vi "create.orderbook.commands.for.testing.vi"(11 "OrderBook.Commands.in":T1[](array[typedef]) {"Side (U8)" format="%.0x"; "Order Id (U64)" format="%.0x"; "Symbol (U64)" format="%.0x"}) -> (3 "Words.Out":u64[](array[numeric]) format="%.0x")   [LabVIEW 2022 SP3]
uses:
  arty/orderbook/orderbook.command.ctl
  arty/orderbook/orderbook.command.type.ctl
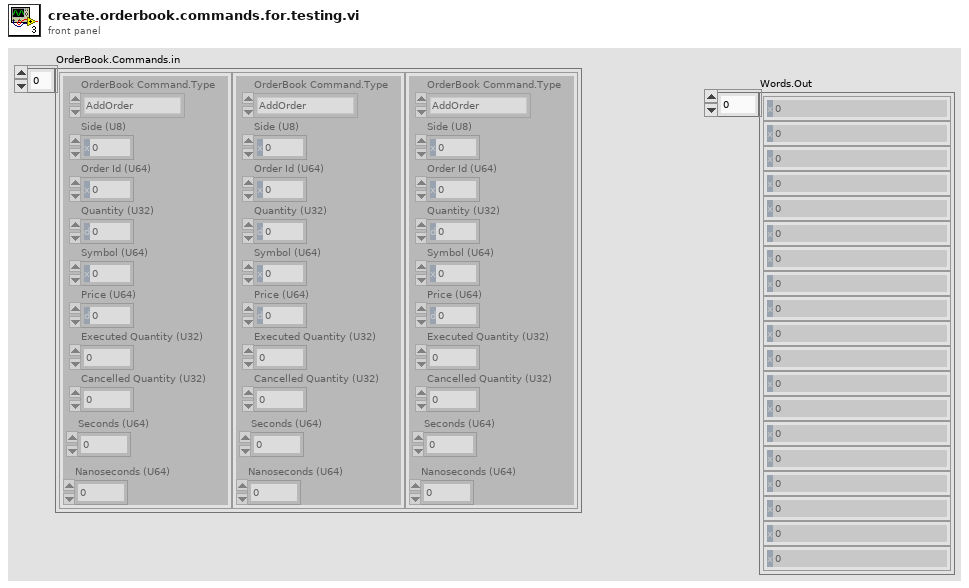
[diagram p1: front panel]
types:
  T1 = typedef "orderbook.command.ctl" = cluster{"OrderBook Command.Type":T2, "Side (U8)":u8, "Order Id (U64)":u64, "Quantity (U32)":u32, "Symbol (U64)":u64, "Price (U64)":u64, "Executed Quantity (U32)":u32, "Cancelled Quantity (U32)":u32, "Seconds (U64)":u64, "Nanoseconds (U64)":u64}
  T2 = typedef "orderbook.command.type.ctl" = enum16{"Time", "AddOrder", "OrderExecuted", "ReduceSize", "ModifyOrder", "DeleteOrder", "Get.All.Orders", "Get.Top"}
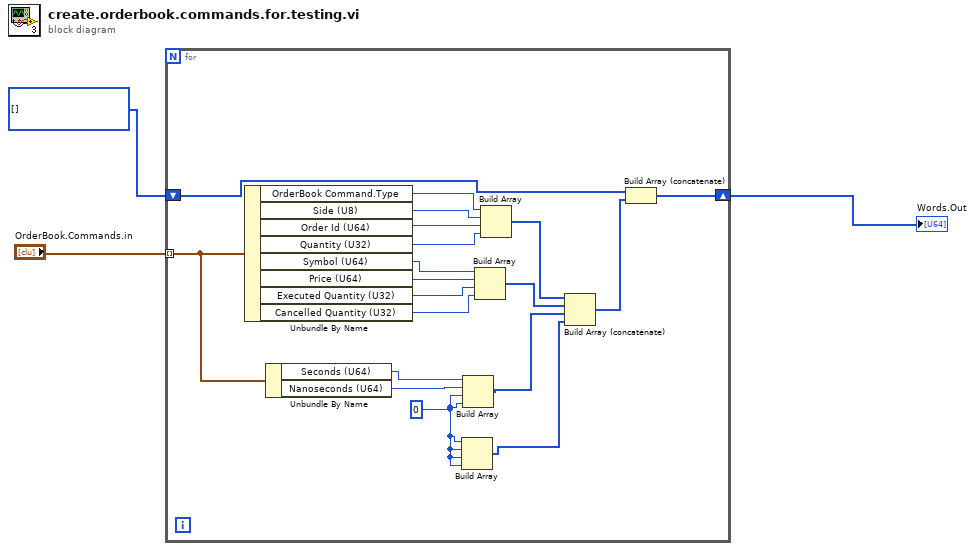
[diagram p0: block diagram]
diagram:
  n1 = for {
    tunnel: "OrderBook.Commands.in" -> [w22] mode=indexing
    shift-right: [w4] -> w1
    shift-left: u64[] [] -> [w6]
    w11 = u64 0 ("element")
    n2 = Unbundle By Name(w22) -> ("OrderBook Command.Type"=w21:T2, "Side (U8)"=w20:u8, "Order Id (U64)"=w19:u64, "Quantity (U32)"=w18:u32, "Symbol (U64)"=w17:u64, "Price (U64)"=w16:u64, "Executed Quantity (U32)"=w15:u32, "Cancelled Quantity (U32)"=w14:u32)
    n3 = Unbundle By Name(w22) -> ("Seconds (U64)"=w13:u64, "Nanoseconds (U64)"=w12:u64)
    n4 = Build Array(w11, w11, w11, w11) -> (w7:u64[])
    n5 = Build Array(w13, w12, w11, w11) -> (w8:u64[])
    n6 = Build Array(w17, w16, w15, w14) -> (w9:u64[])
    n7 = Build Array(w21, w20, w19, w18) -> (w10:u64[])
    n8 = Build Array (concatenate)(w10, w9, w8, w7) -> (w5:u64[])
    n9 = Build Array (concatenate)(w6, w5) -> (w4:u64[])
  }
  "Words.Out" <- w1
